vi "derive weighted array 2.vi"(10 "Full transition sequence from service to end":string[](array[string])=["0 1 0", "0 -1 0", "0 2 0", "0 4 0", "-4 1 0", "0 -4 0", "0 -2 0", "1 0 4", "1 -4 0", "0 -3 3", "0 -3 0", "1 -1 0", "-2 2 0", "0 1 -4", "2 0 -3", "0 -3 3 0", "-1 0 -1", "0 -1 1", "2 -1 0", "0 2 -1", "-3 0 1", "0 1 0 4", "1 0 4 0", "-3 3 0", "1 0 -3", "3 -2 0", "2 0 -3 0", "1 0 -1", "-4 0 -1", "0 -4 1", "2 0 -1", "0 -2 2", "-4 0 -3", "0 -1 1 0", "0 2 0 -3", "3 -3 0", "-4 0 1 0", "-4 1 -4 0", "-4 1 0 4", "0 1 -4 0", "-4 1 -4", "0 2 -1 0", "1 0 3", "0 -3 4 0", "-2 0 2", "1 0 1", "4 0 2 0", "0 2 0 3", "0 -1 2", "-1 0 -4", "1 0 -4", "0 -1 0 -1", "-1 0 2", "-1 0 -1 0", "1 0 -2", "0 -4 0 -1", "0 -2 2 0", "-1 0 1", "2 0 2", "0 1 -1 0", "0 3 -3 0", "-4 0 -2", "0 4 -4", "0 -4 0 -3", "0 4 0 1", "0 -2 0 2", "0 4 0 2 0", "-3 0 1 -4 0 -3", "2 0 1 0", "-2 0 2 0", "0 3 -2 0", "-3 3 0 -2 0", "3 -3 0 1", "-3 0 1 0", "4 -4 0", "0 4 -4 0", "0 -3 3 0 -2", "2 0 2 0", "-2 0 -1", "0 -4 0 1 0", "2 0 -4 0", "2 0 -1 0", "-1 3 -2", "2 0 1", "1 0 -3 3 0", "-4 1 -1", "-4 1 -1 0", "-1 0 -3", "3 -2 2", "-1 1 -1 0", "2 0 4", "1 0 -1 0", "0 -1 2 -1", "0 2 0 -2", "-3 0 -4 1", "0 1 0 -1", "-1 3 0", "0 -1 0 -4", "-2 0 -1 0", "4 0 4", "-4 1 0 4 0", "-4 0 -2 0", "-4 0 2", "0 -2 0 2 0", "0 2 0 -4 0", "2 0 4 0", "4 0 -2", "0 1 0 -4 0", "3 0 1", "2 -2 0", "4 0 -2 0", "0 2 0 4", "1 -4 0 1 0", "0 2 0 -2 0", "-2 2 0 -1 0", "-2 2 0 -1", "-1 0 4 0", "-2 0 4", "-4 1 0 3", "0 -3 0 1", "-2 2 0 -3 0", "0 1 0 3", "0 2 0 1", "0 1 0 1 -4", "0 1 -4 1", "-4 1 0 -3", "1 0 -3 0", "-3 0 -2", "2 -1 0 -1 0", "-3 3 0 -2", "1 0 4 -4 0", "0 -4 0 -3 0", "0 -4 0 1 0 -3 3 0", "0 -3 3 0 2 0 -3 0", "0 -3 3 -3 0", "3 -2 0 1", "-4 0 3", "-2 0 1", "0 3 0", "0 -3 4", "-3 4 0", "-3 0 4", "0 3 -3 0 1 -4 0 -3 3", "0 -2 0 -1", "-4 1 0 -2", "-4 0 -2 0 -1", "-2 0 -4", "0 1 0 -2", "0 -1 0 2 0", "0 -2 2 0 -1", "0 -3 -1 3", "-4 -1 0", "0 -1 2 0", "0 -3 0 -4", "2 0 -3 0 -4", "3 0 -1 1", "-4 1 0 -1", "-1 0 -1 2", "-1 0 -4 0", "0 -4 1 -1", "-3 3 -2", "2 -1 1", "4 -3 0", "1 -4 4", "0 2 0 -1", "1 0 1 0", "4 1 0", "0 2 0 2 0", "-4 0 -1 -3", "1 -4 0 -1", "0 -4 1 -4", "-1 3 0 -4 1 -4", "2 -1 3", "1 -3 0", "-2 0 1 -4", "1 0 -1 1", "0 -3 0 -4 1", "0 2 -1 0 1 -4", "0 -1 3", "0 -4 0 -1 0", "0 4 0 -2", "0 -2 0 -1 0", "0 -3 3 0 -2 0", "0 1 -1 0 -1", "0 -1 0 1 -1 0", "-1 3 -2 2", "-2 2 0 1 0 -1", "0 1 -1", "0 4 0 1 0 4", "-3 0 -4", "1 0 4 0 4 0", "4 -4 0 -2", "4 0 2", "-1 2 0", "1 -1 0 -1", "4 0 1", "2 0 3", "0 2 0", "0 -1 0", "0 1 0", "0 3 0", "0 -4 0", "-2 2 0", "1 -1 0", "0 -2 0", "0 -1 2", "0 1 -1", "0 3 -2", "3 -2 0", "0 2 -2", "-1 0 3", "2 -1 0", "-1 0 -1", "-1 0 -3", "-2 2 -2", "2 0 1", "2 0 2", "0 -3 0", "3 -2 2", "0 1 -1 0", "0 -2 2", "-1 2 0", "2 0 -1", "2 -2 0", "3 -3 0", "0 -1 2 0", "0 -1 0 3", "0 -1 1", "0 2 0 1", "2 -2 2", "0 -4 4", "0 4 0", "2 0 3", "-2 3 -2", "2 -2 3", "4 -4 0", "0 1 0 -3", "0 3 0 3", "-1 0 4", "-3 0 -2", "-4 0 -2", "2 0 2 -1", "-1 0 2", "-2 0 -1", "-4 4 0", "0 2 0 -2", "-1 1 -1", "-1 1 -1 0", "-2 0 -2", "3 0 -4 0", "3 0 3", "0 1 0 3", "0 3 -3 0", "2 0 -2", "3 0 -2", "0 -3 3", "3 -2 2 -2", "-3 0 -2 0", "1 0 -3 0", "-1 0 2 0", "3 0 -4", "-1 0 1", "-1 0 -1 0", "0 -1 2 3", "-1 3 -2 0", "3 -1 3", "-2 0 2 0", "0 1 0 -3 0", "0 -4 0 -2", "1 4 -4", "0 -2 2 0", "1 4 0", "0 3 -2 0", "-2 0 -4 4", "-1 0 3 0", "0 2 0 -1", "0 2 -2 3", "4 0 -1", "-1 2 0 2", "1 -1 0 -3", "-2 0 2", "2 0 -4", "0 3 -2 2 -2 2", "0 2 -2 0", "4 0 -4 0", "0 3 0 3 0", "4 -3 0", "-3 4 -3 0", "0 4 -4", "3 0 -1", "-2 2 -2 0", "0 -2 3", "-2 0 3", "1 0 -3", "2 -2 2 0", "0 -3 4", "0 -1 1 -1", "0 4 1 4", "1 -1 0 -1", "1 4 -4 0", "-4 0 2 0", "-4 0 2", "0 -2 2 3 0", "0 -1 1 -1 0", "0 2 0 1 4", "4 0 1 0", "2 3 -2", "0 -1 2 3 -2", "0 -1 0 4", "-4 0 1", "-1 0 -1 2", "-2 0 -1 0", "0 3 0 -1", "3 -2 0 -1", "0 -4 0 -2 0", "2 0 -4 0", "0 -2 0 2", "-1 0 -3 0", "0 -3 0 -2", "2 0 -1 0", "0 -1 2 0 1", "0 -2 0 -4 4 0", "0 -4 4 0", "-1 -3 0", "0 -2 0 3", "2 0 -2 2", "-4 1 0", "-1 1 4", "-1 0 3 -2", "0 2 0 4", "0 -4 4 0 -1", "3 0 -2 0", "0 3 0 -2", "2 0 1 -1 0", "0 1 -1 0 2 0", "0 2 0 1 -1", "2 0 -1 2", "-2 3 0", "0 -1 0 2", "0 1 -1 0 -3", "2 0 1 -1", "-2 0 -1 2", "-1 4 0", "0 -4 1", "2 0 2 0", "2 -1 1", "4 -4 0 -1", "-4 0 -1", "-1 0 4 0", "2 0 2 -1 0", "0 -3 3 0", "-1 0 -3 3", "-1 0 1 -1 0", "0 3 0 -4", "-2 2 -2 0 -2", "-2 0 4 0", "0 1 0 3 0", "4 -3 0 -2 0", "0 3 -2 3", "2 0 3 -2", "3 -2 3", "0 2 -2 3 -2 2", "-2 2 0 3", "3 -2 2 0", "3 -2 2 0 3", "3 -2 3 -2", "0 -3 4 -3 0", "0 -1 0 -3", "3 -3 0 1 0", "0 2 0 3", "0 3 -2 2 -2 2 0", "0 2 0 2", "-2 3 -2 0", "4 0 -2", "-4 0 -1 0 3", "-2 2 -2 3", "0 -1 0 -1 0", "-2 2 0 3 0", "0 2 -2 2", "2 3 -2 2 0", "-2 2 -1", "-4 0 -2 2", "0 -4 0 2", "-1 2 -1", "-1 0 3 -1 3 0 -4", "-1 3 -2", "4 0 -4", "3 0 3 0", "0 3 0", "0 1 0", "0 2 0", "0 4 0", "0 4 -4", "0 -3 4", "0 -3 0", "0 -4 0", "0 3 -2", "0 -1 0", "-4 1 0", "1 0 3", "0 2 0 -3", "2 0 3", "3 -3 0", "-3 0 3", "0 -3 3", "0 -3 4 -3 0", "0 -2 0", "3 -2 0", "0 3 0 1 0", "0 -3 4 0", "2 -2 0", "-2 0 -3", "4 0 2", "-3 0 2", "0 3 -3 0", "4 -4 0", "0 -1 2", "3 0 4", "0 3 -2 0", "0 -3 0 3", "1 0 -1", "0 4 -4 0", "-2 0 3", "0 2 -2 0", "0 2 0 -3 4", "3 -3 0 -3", "4 0 2 0", "3 0 -2", "0 -3 3 0", "-1 0 3", "0 -1 2 0", "-4 0 -1", "2 0 3 0", "0 3 0 3", "-4 0 3", "0 4 -4 1", "4 0 -3", "0 -1 0 4", "0 3 -3 0 2", "0 -2 0 3", "0 -3 4 0 3 0", "-3 0 4 0", "0 3 0 3 0", "0 4 0 -3 0", "-3 4 0", "2 0 -3 4", "0 2 0 -3 4 0", "0 1 0 2", "0 -2 3", "-2 0 -2", "0 -3 4 0 2", "0 -3 3 0 -2 2", "1 0 -3", "0 -1 1 0", "4 -4 0 -4", "-4 0 3 0", "2 0 -3", "-2 0 3 0", "0 4 -4 1 0", "-4 1 0 -1 2 0", "3 0 4 -4", "0 -3 4 -3 0 2", "3 0 3", "-1 0 -3", "-3 4 -3", "4 -3 0", "0 -3 4 -3", "-3 4 -3 0", "4 0 2 0 3", "0 2 0 3", "-4 1 0 -4 0 4 -4", "-4 1 -1", "-1 0 -4 0", "1 0 3 -2", "0 -1 0 3", "0 3 0 4 0", "0 2 0 3 0 1 0", "-4 1 -4 1", "1 -4 1 0", "0 -4 4", "0 1 0 4", "1 -4 1", "-3 0 1", "0 4 -4 0 -1 0", "-3 0 4", "2 0 -3 4 0", "1 0 2", "4 -3 0 2", "-3 4 -3 0 2", "3 0 1", "1 -1 0", "0 -1 0", "0 1 0", "0 1 -1 0", "0 4 0", "0 3 0", "-1 0 4", "-1 0 -3 3", "1 0 1", "-4 1 -1", "0 4 0 2", "0 -1 0 -3", "3 -2 2 -1 0", "2 -1 0", "0 1 -1", "-1 0 3", "-1 1 -1 0", "-3 0 1", "-1 0 3 0 -4", "-1 0 -3", "1 -1 0 -3 3", "1 -1 0 3", "2 -1 0 4 -4", "1 0 1 0", "0 -1 0 4", "2 0 3 0 -1", "-4 1 -1 0", "0 3 0", "0 -1 0", "0 4 0", "-1 0 3", "0 -3 4", "0 -3 3", "1 -1 0", "0 3 -2", "0 2 0", "0 1 -1", "4 -3 0", "-4 0 -3", "0 -4 0", "4 0 2", "0 1 -1 0", "0 1 0", "0 4 -4", "3 -2 2", "2 -1 0", "0 -2 0", "0 -3 4 0", "-1 0 -3", "0 3 -2 0", "0 -3 3 -3 0", "0 -3 4 -3 0", "4 0 4", "0 1 -1 0 3", "3 -2 2 0", "-2 2 0", "3 0 1", "0 4 0 2", "0 2 -1", "2 0 4", "-1 0 4", "0 -3 3 0", "-1 0 1", "-1 0 -1 0", "-1 0 -1", "4 -3 0 2", "0 -3 0", "-4 0 -3 0", "-3 0 3 -2", "0 3 -2 2 0", "-4 0 -3 3", "0 3 0 -4", "2 0 4 -4", "0 2 0 4", "0 4 0 -4", "2 -1 0 1 -1 0", "0 2 -1 0", "-1 0 -3 3", "0 -4 4 0", "0 4 -4 0", "-4 0 3 0", "0 -2 3", "-3 0 -3", "0 -2 0 -3", "-3 0 1", "-2 3 0", "0 3 0 -2", "0 4 -3 0", "4 -3 0 2 0", "0 -3 4 -3 0 3 -2 2 0", "3 0 -3 4 -3 0", "-1 0 3 -2 3", "-1 0 3 -2", "0 1 0 3", "1 0 3", "4 -3 0 -2", "-4 0 -3 4", "-2 0 3 0", "2 0 2", "0 2 0 2 0", "-4 4 -3 0", "0 -4 0 -3", "3 0 3 0", "-4 0 -3 3 0", "4 0 3", "0 4 0 4", "4 0 4 0", "0 4 0 -4 0", "0 -1 0 -2", "4 0 2 0", "1 0 -3", "0 -4 1 -4", "0 4 -4 0 -3", "-2 2 0 4 -4", "0 4 -4 4 -4", "4 0 2 -2", "0 4 0 -2", "0 3 0 1", "4 -4 1", "4 0 2 -1 0", "0 -4 4 0 2", "-1 0 3 0", "0 3 -2 0 -1 0", "1 -1 0 4", "0 4 0 1", "-1 0 4 0", "1 0 3 -2 0 -1 0", "0 -4 0 3 0 -4", "-1 0 -4", "1 -4 0", "1 0 4 0", "0 -1 0 -1 0", "-1 0 -3 3 0", "0 -1 0 -1 0 -3", "-2 2 -1 0", "0 -1 0 3 -2", "2 -1 0 1 -1 0 3", "-2 3 -2 2 -1", "-2 2 -1", "0 -1 0 4", "3 0 1 0", "0 3 -2 0 -1 0 -1 0", "-3 4 0", "3 0 -1", "0 4 -3", "3 0 3", "-4 0 3", "4 -4 0", "0 -1 0 -1", "0 3 0", "0 -3 4", "0 -3 3", "0 3 -3 0", "0 2 0", "4 -3 0", "0 3 -3", "0 3 -2", "0 -3 4 -3 0", "-4 0 -3", "3 0 -3", "0 -4 0", "-3 0 -3", "0 -3 3 0 3", "0 -3 3 0", "0 -2 0", "-3 0 3", "3 -3 0", "3 0 3", "-3 4 0", "-4 0 -3 4", "-3 0 4", "0 -1 0", "3 0 -3 3", "-3 3 0", "0 3 -2 0", "0 -3 4 0", "1 0 -3 4", "0 -3 0", "0 -1 0 -3", "-3 0 3 0", "-2 0 3 -2", "0 1 0", "0 -2 0 3", "-2 0 -3", "0 3 0 -3", "3 0 3 -3", "3 -3 0 3", "-3 0 -3 3 0", "0 -3 4 -4 0", "0 2 0 -2", "-2 0 3", "0 3 -2 3 0", "-2 3 0 -3 3", "3 0 -1", "-3 0 -4", "1 -1 0", "-4 0 -2", "0 3 -3 0 4", "-2 3 0", "-1 0 3 -2", "-3 4 -3", "0 -3 4 -3", "-3 4 -3 0", "-3 3 0 3", "-2 0 2", "0 -1 0", "0 -2 3", "3 -2 0", "-2 3 -2 0", "0 2 0", "0 1 0", "0 4 0", "2 0 -1 0", "0 3 -2", "2 -2 3", "-2 0 2", "0 2 -2 0", "4 -3 0", "-3 0 -2 0", "0 3 0", "0 -3 -2", "-2 3 -2 0 3", "0 3 0", "0 -2 0", "0 1 0", "0 3 -2", "2 -2 0", "0 2 0", "3 -2 0", "0 -3 4", "0 4 0", "-2 0 -2", "0 -3 0", "3 -2 2", "1 -1 0", "0 2 -2", "-2 3 -2", "0 -1 0", "0 -4 0", "0 2 -2 0", "-1 0 3", "0 -2 3", "2 0 -2", "0 3 -2 0", "0 -3 4 0", "-3 0 3", "0 3 -3", "4 -3 0", "-2 0 -3", "0 -2 3 -2", "-2 2 0", "0 3 -2 2", "3 -2 2 0", "2 0 2", "3 -3 0", "2 0 3", "0 -2 0 -2", "-3 4 0", "0 3 -3 0", "-1 0 3 0", "-2 0 1", "2 -1 0", "0 -3 4 -3", "0 3 -2 2 0", "-2 0 1 0", "-3 0 4", "0 -2 2", "-2 3 -2 0", "0 3 -2 3", "0 1 -1 0", "1 0 1", "0 -3 0 3", "0 -3 3", "3 0 -3", "0 -1 0 3", "4 0 1 0", "0 -2 3 -2 0", "2 0 3 -2 0", "0 2 -1", "3 -3 0 4 0", "-2 0 -4", "-3 0 -2", "3 0 3", "0 3 0 3 0", "0 3 -2 3 -2", "-2 3 -2 2", "-3 0 1", "-2 0 3", "-2 0 -3 0", "0 3 -2 2 0 2", "2 0 2 0", "1 -1 0 3", "0 3 -2 0 -2 2", "-2 0 -2 2", "2 0 -2 3 -2", "1 0 -2", "1 0 3", "2 0 -4 0", "-1 0 1", "0 2 0 4", "4 0 -2", "0 -2 0 1", "0 -1 0 3 0", "0 2 0 3 -2 0", "0 3 -2 0 1 0", "-1 0 -1 0", "-2 2 0 -2", "2 0 -2 0 -2", "0 4 0 1 0", "0 1 0 4 0", "0 1 0 -3", "0 -3 0 3 -2", "1 0 -3 0", "4 0 -4 0 1", "-1 0 -4", "0 -3 3 -3 0 4 0", "0 -4 0 3", "0 3 0 2", "1 0 1 0", "0 4 0 3", "1 -1 0 -3 4 0", "3 -2 0 -4", "2 -1 2 0", "-4 1 0", "3 -2 0 -4 0", "-2 0 -3 4", "0 -3 4 -3 0", "0 -2 0 -3", "-2 0 -3 4 -3 0", "2 -2 3", "0 2 -1 0", "2 0 2 -2 0", "0 -3 4 0 2", "1 0 2", "-3 4 0 2 0", "-2 0 -4 1", "0 3 -2 0 -4", "0 2 0 2", "-2 3 0", "1 0 -3", "0 3 0 -3 4", "-3 4 0 2", "-2 0 -2 2 -2 0", "2 -2 0 -3 4", "0 -3 4 -3 0 3", "4 -3 0 3 0", "3 0 -2", "0 -2 0 -2 0", "4 -3 0 3", "0 4 -3 0", "-3 0 -2 0", "-1 0 -1", "1 0 4", "2 0 2 -2", "-2 0 -2 0", "1 -1 0", "-1 0 1", "0 1 0", "0 -1 0", "0 1 -1", "-1 0 -1", "0 4 0", "2 -1 0", "-1 0 1 -1", "-1 0 4", "0 -3 0", "0 1 -1 0", "-1 1 -1", "-1 0 -3", "-1 0 -1 0", "0 -1 0 1", "1 -1 0 -1", "-1 1 -1 0", "1 -1 1", "4 0 2", "0 1 -1 0 1", "1 -1 0 4", "0 1 0 -4", "0 4 -4", "-1 0 -1 0 1", "-1 0 4 0", "0 1 -1 1 -1 0", "1 0 -4 0", "1 0 -4", "0 4 0 -1 0", "-1 0 1 0", "0 4 -4 0", "-1 0 -3 4 0", "0 1 0 -1 0 -3", "0 1 0 -4 0", "-4 0 4", "0 -1 1 -1", "-2 2 -1 0", "0 -3 0 -1 0", "2 -1 0 -3", "-1 0 3 0", "-1 0 -3 0", "-1 0 -2", "0 2 0", "1 -1 0 4 0", "-1 0 4 0 -1 0", "0 1 -1 1 -1 0 4", "0 -2 2 -2", "-1 0 -1 0 1 0", "3 0 1 0", "0 4 0 1 -1", "1 -1 0 1", "0 1 -1 1", "1 -1 1 -1", "0 1 -1 1 -1", "1 -1 1 -1 0", "0 -1 1", "0 -4 0", "-3 0 -1", "4 0 -1", "-1 1 -1 0 4", "1 -1 1 -1 0 4", "-2 2 0", "1 -1 0", "0 1 0", "0 -1 0", "3 -3 0", "0 3 0", "0 1 -1", "0 4 0", "0 2 0", "2 -1 0", "-1 0 1", "0 -2 0", "-4 1 0", "1 0 1", "0 1 -1 0", "-1 0 -3", "-1 0 4", "0 4 0 -2", "0 4 -4", "-1 0 1 0", "0 3 -3 0", "0 -4 1", "0 4 -4 1", "-4 4 0", "-1 0 3", "0 -2 3", "0 -3 4", "1 0 1 -1", "-2 0 -3", "0 -3 0", "0 -3 3", "-2 3 -3 0", "1 0 -2", "-2 3 -2", "4 -4 1", "1 -1 0 4 -4 1", "-1 0 4 -4 1 -1", "-4 1 0 1 -1 0", "0 1 0 -4", "0 1 0 -2", "-1 0 -1 0", "2 -1 0 1", "1 -1 0 1 0", "3 -2 0", "0 -2 2", "2 0 2", "3 -3 0 1", "-3 0 3", "-2 2 0 -3", "0 3 -3", "-3 0 -4 4", "0 4 0 -2 3", "0 -4 4", "-1 0 3 0", "4 -4 1 0 4", "4 0 1 0", "1 -1 0 -3", "-2 0 1 -1", "0 4 -4 1 0", "0 -4 4 0 1", "1 0 -2 3 -2", "1 0 4", "0 -4 1 0", "0 1 0 -4 1 0", "-2 0 1", "4 -3 0", "-3 0 4", "0 4 -3 0", "1 -1 0 4 -4 1 -1 0", "4 -4 1 0", "1 0 4 0", "1 -1 0 -1 0", "0 -4 0", "4 0 1", "0 1 0 1 0", "2 0 4 0", "0 -2 0 2 0", "2 0 1", "-1 0 -3 4", "4 0 2 0", "0 -2 0 1", "-1 0 4 -4 1", "3 -2 3", "3 -2 2 0", "1 -1 0 3", "-1 0 -1", "0 -1 1", "-1 0 1 0 3", "0 -4 1 0 1 -1 0", "0 3 -2", "0 1 0 3", "1 -4 0", "0 -2 2 0", "1 -1 1 -1 0", "0 1 0 3 -3 0", "-3 0 -3 3", "0 -3 3 0", "0 3 0 -2 0", "0 2 0 2", "-4 0 -2", "3 0 3", "3 0 3 0", "0 -3 3 -2", "0 2 -2 3 -3 0", "-2 2 0 -3 3", "-3 0 1", "3 -3 0 3", "0 3 -3 0 1", "0 3 0 2", "2 0 -3", "-2 3 -3", "3 -2 2", "-4 1 -1", "2 0 -3 3", "0 4 0", "0 -2 0", "1 -1 0", "-1 2 -1", "0 2 0", "2 -1 0", "0 3 0", "0 -1 0", "-2 0 3", "0 -4 0", "3 -2 0", "0 3 -2", "0 -3 0", "-1 0 3", "0 -2 0 3", "0 1 -1 0", "0 3 -2 0", "1 -4 0", "-1 0 2", "0 -1 2", "2 0 3", "0 -3 3", "3 -3 0", "3 0 -1 0", "-2 0 -2", "2 -2 0", "-3 3 0", "0 2 0 3", "0 1 0", "0 -2 2", "-4 0 -1", "0 -1 2 -1", "-1 0 -1", "2 -1 2", "-1 3 -2", "3 0 -4", "3 -2 2", "-1 1 -1 0", "-1 2 -1 0", "0 1 -4", "4 -4 0", "2 -3 0", "0 3 0 -2", "2 0 3 0", "0 1 0 -3", "1 0 -3", "-1 0 -4 0", "-4 0 1", "2 0 -2 0", "-1 0 -3", "0 -3 4", "4 0 1", "0 1 -4 0", "0 -1 0 3", "0 -3 3 0", "0 3 -3 0", "0 4 0 2", "0 2 -2 0", "-2 0 -3", "3 0 3", "-1 0 -2", "-2 0 3 0", "2 0 4 0", "0 4 0 -2 3", "0 -3 0 -2", "-3 0 -2 2", "1 0 4 0", "-3 0 2", "0 -2 0 3 -2 0", "1 0 -3 0", "-3 0 -2", "-2 0 -2 0", "0 4 -4", "-1 -3 0", "-2 2 -1", "2 0 -3", "-1 1 0", "2 -1 1", "-2 2 0", "0 -4 0 -1", "0 -1 3 -2 2", "-1 2 -1 2", "-1 2 0", "-1 3 0 -1 0", "2 0 2", "-1 0 2 -3 0", "-1 0 2 0", "-1 4 -4 1", "-1 0 4", "2 -1 0 -1", "2 -1 0 2", "-4 1 -1", "3 0 -4 1", "1 -1 -3 3", "0 1 0", "0 -2 0", "1 -1 0", "0 3 0", "0 2 0", "0 3 -2", "3 -2 0", "0 -4 0", "-1 0 -2", "-2 2 0", "0 -1 0", "1 -1 0 -2", "0 -2 2", "-2 0 -2", "0 1 0 1", "4 -4 0", "0 3 -3", "0 1 -1", "1 0 1", "0 3 -2 0", "-2 2 -2", "0 -2 3", "0 3 -3 0", "0 4 0", "2 0 3", "0 -2 3 -2", "0 4 -4 0", "-2 0 -2 0", "1 -1 0 -2 0", "-2 0 2", "-4 0 -4", "0 -4 0 1", "0 2 0 -4", "3 0 -2", "-1 0 3", "0 1 -1 0", "-3 0 -1", "-1 0 2 0", "4 -3 0", "1 0 -2", "0 1 0 1 0", "0 -2 3 -2 0", "3 -2 0 -2 0", "0 -2 2 -2 0", "0 -2 0 -2", "-1 4 0", "4 0 2", "1 -1 0 -2 0 2 0", "2 0 -2", "-2 0 4", "0 -1 0 3", "0 -2 2 0", "1 0 3", "0 1 0 3", "4 0 -2", "0 -4 0 -4", "0 2 0 -4 0", "-4 0 -4 0 1 0", "-1 2 3 0", "3 0 3", "0 -4 0 3 0", "2 0 1", "2 -1 0", "-1 0 -1", "-2 3 0 -2", "3 0 -2 0", "0 1 -1 0 -2", "0 3 0 -2", "3 -2 2 -2", "1 0 1 -1", "0 4 -3 0", "2 0 -1 0", "0 2 0 3", "2 0 3 0", "2 0 -3 4 -3", "-2 2 0 -3 4", "2 0 -3 4", "0 3 -3 0 -1 0", "1 0 4", "0 3 0 1", "1 0 3 -2 0", "-2 3 0", "1 0 1 0", "0 4 0", "0 2 0", "0 3 0", "0 -3 0", "0 1 0", "-4 0 -3", "0 -4 0", "0 3 -3 0", "0 -3 0 3", "-4 0 3", "0 4 0 2", "0 -3 3", "-4 0 -3 0 3", "0 2 0 3", "-3 0 2", "0 4 0 1", "0 -4 0 3", "0 4 0 2 0", "0 -2 0", "0 1 0 4", "4 0 2", "0 4 0", "0 3 0", "0 2 0", "4 -4 0", "0 4 -4 0", "0 -2 0", "3 -3 0", "0 4 -4", "0 3 -3", "0 3 -2", "0 4 0 2", "4 0 2", "0 1 0", "0 3 -3 0", "0 -3 0", "2 -1 0", "0 -1 0", "1 0 3", "4 0 3", "3 -2 0", "0 1 -4", "-1 0 4", "0 -4 0", "0 -3 3", "2 0 4", "-4 1 0", "0 -2 2", "0 4 0 3", "-1 0 1", "0 3 -2 0", "-3 0 4", "-1 0 3", "0 -3 4", "0 4 0 -2", "1 -1 0", "2 0 4 0", "0 -4 4", "0 -1 0 4", "-1 0 4 0", "4 -3 0", "0 2 -1 0", "1 -4 0", "2 0 -4", "-2 0 4", "0 4 0 2 0", "3 0 3", "0 -3 3 0", "2 -2 0", "1 0 -3", "-4 0 2", "1 0 3 0", "0 1 0 3", "-1 0 3 0", "3 -2 2", "-4 1 -1", "2 0 -3", "0 -4 1", "0 2 0 -4", "-3 0 4 0", "3 0 -2", "0 -2 2 0", "0 -2 3", "-4 0 2 0", "0 3 0 -4", "0 2 0 4 0", "-2 0 2", "-2 2 0", "0 3 0 4", "-3 4 0", "-1 0 1 0", "4 0 4", "0 1 0 3 0", "0 -1 0 4 0", "0 3 0 3", "1 0 -3 0", "0 3 0 1", "-2 2 -1 0", "0 3 -2 2", "-3 0 2", "1 -1 0 3 0", "0 3 0 -2", "-4 0 -4", "0 1 0 -3 0", "0 4 0 -3", "2 -1 0 4", "1 -4 1", "-4 0 3", "-2 0 -4 0", "0 3 -3 0 4", "-4 0 -2", "0 4 -4 0 3", "0 -2 3 -2 0", "0 4 0 4", "-1 2 -1", "-3 0 -2", "-3 0 -3", "-4 0 4", "4 0 -3", "3 0 -4", "2 0 -2", "-2 0 2 0", "0 -4 4 0", "0 2 0 3", "-2 0 1", "4 0 3 -3 0", "0 -2 0 3", "0 4 0 3 0", "0 2 -2 0", "2 -2 0 4", "4 0 -2", "2 0 -1", "0 1 -4 0", "0 -1 2", "4 0 -1", "0 1 -4 1", "4 -4 1", "0 3 -2 0 1", "4 0 4 0", "0 -1 0 4 0 4", "1 0 4", "0 1 -4 1 0", "0 4 0 2 0 -3", "-2 0 4 0", "0 2 -2 0 4 0", "0 -3 0 2", "-4 0 -2 0", "0 -2 0 2 0", "0 2 0 -1", "0 -1 3", "0 -4 4 -4", "3 -2 0 -4 0", "-4 0 -1", "-3 0 3 0 3", "-1 0 3 -3 0", "-3 0 3 0", "0 3 0 3 -2", "-2 2 -2", "-1 0 1 0 3", "-2 2 -1 0 1 0", "0 2 -1 0 -3", "0 4 0 2 -1 0", "-1 0 4 -4 0", "0 2 -1 0 4 -4", "0 4 -4 0 3 -2 0", "-1 0 -3", "-2 0 1 -4", "0 3 0 4 0", "0 1 -4 4", "-1 0 -3 0", "-1 0 4 -4", "0 4 0 -2 0", "0 4 -3 0", "4 0 -3 3", "-1 0 -2", "0 -2 0 3 -3", "1 -4 1 -1 0", "-4 1 -1 0", "-2 0 -2 2", "0 -1 2 -1", "-4 0 -4 1", "0 2 0 4 0 2 0", "0 3 0 -1", "3 0 3 0", "0 -3 0 3 0", "0 3 0 4 -4 1", "-1 0 -4", "0 -4 1 0 3 0", "0 2 -1", "-4 0 4 0", "0 -2 0 4", "0 4 0 -1", "-4 0 3 0", "0 3 0 -2 0", "0 -3 4 -3 0", "-4 0 2 0 -4", "2 0 -2 0", "-2 2 0 -3", "3 0 2 0 4 0", "3 0 2 0", "1 -4 0 2 0", "3 0 -4 4 0", "3 0 -4 4", "3 -3 0 4", "-2 3 -3", "0 -4 0 2 0", "0 3 0 -4 0", "3 -3 0 4 0", "0 3 -3 0 4 0", "4 0 3 -2", "-4 0 -3", "-3 0 -3 4", "3 -3 4 0", "1 -4 -1", "-3 3 -3 0", "0 -1 1", "-3 0 4 0 3", "0 3 -3 0 -2", "0 4 0 3 -3 0", "4 -3 0 4", "0 3 0 2 0", "0 4 0 -2 2", "-4 -1 0 1", "-1 0 1 0 -3 0", "-3 0 1 -4 0", "-3 3 0", "0 -1 0 1", "-1 0 1 -4", "0 3 0 -4 4", "-4 1 -1 0 3 0", "0 1 0 3 0 1", "-3 0 3", "4 0 -2 0", "4 0 2 0", "3 0 -1", "4 0 3 -3", "3 -3 0 -2", "3 0 4", "3 0 2", "2 0 3", "4 0 -2 2", "-2 2 -1", "0 2 -1", "0 4 0", "2 -1 0", "0 -4 0", "0 2 -1 0", "3 -2 0", "4 -3 0", "0 -1 2 0", "0 -1 0", "0 2 -2", "-4 0 1", "-4 0 -4", "0 -4 0 -4 0", "-1 0 4 0 2", "-2 2 0", "1 0 -4 0", "3 -2 2", "0 2 3 -2", "2 -1 0 2 -1", "2 -1 -3", "3 -2 0 -4", "0 -3 4 -3 0", "-1 1 -1 0 -1", "0 -4 1 0", "-1 0 2", "4 0 2", "0 2 0", "0 1 0", "0 -4 0", "0 -2 0", "0 2 -2", "2 -2 0", "0 4 0", "0 3 0", "0 2 -2 0", "0 -1 0", "0 -3 0", "-4 0 -2", "-2 0 2", "1 0 4", "-2 0 -4", "0 3 -2", "3 -2 0", "1 -1 0", "-2 3 0", "0 -1 2", "0 -3 4", "4 -3 0", "-2 0 4", "0 4 -3", "-2 0 -4 0", "-2 2 -2", "3 0 1", "4 0 2", "-1 0 -1", "0 -2 3", "1 0 -4", "-1 0 -1 0", "-2 0 -3", "1 0 -3", "-2 0 3", "2 0 -2", "-2 2 -2 0", "-4 0 -2 0", "0 1 0 4", "0 3 -3", "2 0 1", "1 -4 0", "0 -4 1", "0 3 -2 0", "-3 4 0", "0 -4 0 -2", "2 -1 0", "0 3 0 1", "0 1 -4 0", "3 0 2", "-3 0 -4", "-4 0 2 -2 0", "0 -4 0 2 -2", "2 0 -2 0", "0 4 -3 0", "-4 0 2", "-4 0 2 -2", "-2 2 0", "-4 1 0", "0 4 -4", "-2 0 2 0", "0 -2 0 2", "1 0 3", "-2 0 4 0", "2 0 -4", "-2 3 -2", "0 2 0 1", "0 4 0 2", "0 2 -2 2", "0 1 -1", "0 -4 0 -3", "-1 0 -4", "-1 0 -2", "2 -2 0 -4 0", "2 0 3", "0 -4 0 2", "0 -3 4 0", "0 3 -3 0", "0 -4 0 -2 0", "-2 0 -2", "0 -3 3", "0 -2 0 -4", "0 -4 1 0", "4 0 2 -2", "-3 0 -4 0", "0 -3 4 -3 0", "2 -2 0 2", "0 1 0 -1", "2 -2 0 4 0", "2 -2 0 4", "1 0 -4 0", "-3 0 3 0", "0 3 0 -2", "2 -2 3", "0 2 0 -2 0", "0 1 0 3", "1 0 4 0", "-4 4 -4 0", "-2 0 1", "0 -4 0 3 0", "1 0 1 0", "-1 0 3", "0 -1 2 -1", "0 -1 0 -1", "0 4 0 3", "0 -2 0 4", "0 -4 4", "0 3 0 1 0", "1 0 -3 3", "0 2 -1", "-1 0 1", "-2 0 -3 0", "1 -1 0 -2", "-1 0 -2 0", "3 0 3", "-1 1 0", "3 0 -2", "3 0 4 0", "0 2 -2 2 -2 0", "0 1 0 -4", "0 2 0 4 -3", "-2 0 -2 0", "0 3 0 -2 0", "-2 0 -2 3", "0 2 0 3", "0 -2 0 2 0", "0 -3 3 0", "4 0 -3", "0 1 0 -3", "1 0 4 -3 0", "2 -2 0 -2", "0 -1 1", "-1 1 -1 0", "0 1 0 -1 1", "0 -3 0 -3", "-1 0 -3", "4 -3 0 1", "-3 4 0 2", "0 2 -2 0 -3 4", "3 -2 0 -3 0", "0 -2 0 3", "-2 0 -4 0 2", "0 2 -2 0 -4 0", "0 -2 0 4 0 3", "4 0 -2 0", "0 -4 0 -3 4", "0 1 0 -4 0", "0 -2 2", "0 4 0 4", "2 0 -4 0", "-4 0 -1 2", "3 0 3 0", "0 3 0 2", "0 2 -1 0", "2 -2 3 0", "0 1 -1 0", "0 1 0 4 0", "0 1 -4 0 -2", "0 -2 0 2 -2 0", "0 -2 0 -3", "-4 0 1", "-2 0 2 -2 0 3 0", "-2 0 3 0 1 -4 0", "4 -1 0", "0 2 -2 0 2", "2 0 2 -2", "1 0 -4 4", "-1 0 4", "2 -1 0 -4 0 -3", "0 -1 2 -1 0", "-1 0 3 0", "-3 0 3 0 1 0", "1 -4 0 -4", "0 1 0 -2", "-2 0 -4 0 3 0", "0 4 0 2 -2 2 -2 0 -4 0 3", "0 2 -2 0 4", "-2 0 2 -2 0", "0 -1 1 0", "1 -1 0 -2 0", "0 -4 0 3", "4 0 1", "-2 0 -1", "-1 0 -1 0 -1", "0 1 0 3 0", "-1 2 0", "-1 0 1 0", "3 -2 3", "0 -2 3 0", "3 0 2 0", "0 3 0 4 0", "-1 0 2", "0 -3 0 -1 0", "-4 0 -3", "-1 0 -2 3", "0 -2 3 -2", "0 -2 3 -2 0", "-2 0 -4 0 3", "0 3 0 3", "0 -2 0 -4 0", "0 4 0 -4 0", "1 0 2", "3 0 -2 3 -2", "-3 0 2 -2 0", "4 -3 0 2", "-3 0 -2 0", "2 0 4", "0 2 0 4", "2 0 4 -3", "0 2 0 4 -3 0", "-3 0 2", "-3 0 -3", "4 0 4", "1 0 -2", "-2 0 2 -2", "1 0 1", "2 0 4 -3 0", "-3 0 3", "3 -3 0", "0 3 0", "-3 3 -3 0", "-3 3 -3", "0 -3 3 -3", "0 -3 3 -3 0", "2 -1 0", "0 -3 3", "-3 0 -3", "3 -3 0 -3", "-3 0 -3 3", "0 2 -1", "0 1 0", "0 3 0 3", "0 -1 0", "3 -3 0 -3 3", "0 2 -1 0", "0 4 0", "0 3 -2", "-1 0 2", "3 -2 0", "0 -4 0", "0 -3 0", "3 0 2", "0 3 -3", "0 -3 4", "-3 0 -3 3 -3", "0 3 -2 0", "-1 0 4", "-1 0 3", "-1 0 3 0", "0 1 0 3 0", "1 0 -1", "0 1 0 -1 0", "3 0 1", "0 2 0", "0 -1 2 0", "-3 0 -2", "3 0 -3", "0 -2 3", "0 -3 3 -3 0 -3 3", "3 0 3", "0 2 -1 0 2", "0 2 -2", "2 -2 3", "1 -1 0 3", "0 3 -2 0 1 0", "0 4 0 -1", "0 1 -4", "2 -1 0 4", "0 4 -4", "0 1 0 3 0 1 0", "1 0 3", "0 1 0 3", "1 0 3 0", "2 0 -1", "0 -1 0 3 0 3 0", "0 2 0 3 0", "2 0 4 0 2", "-4 0 -3", "4 -4 0", "0 3 0 3 -3", "-4 0 3 0", "0 -3 4 -3", "-3 3 0", "-2 0 3", "0 -2 0", "1 0 -3", "2 -2 0", "3 0 -3 4", "-3 0 -3 3 -3 0", "3 -3 0 -3 3 -3 0", "0 -3 3 -3 0 -3 3 -3 0", "0 3 0 -3", "-3 3 -3 0 -3", "0 -3 3 -3 0 -3", "-3 3 -3 0 -3 3", "2 -1 0 2", "3 0 3 0", "2 0 3", "3 -3 0 -3 3 -3", "0 3 0", "0 2 0", "0 4 0", "0 -3 4", "0 1 0", "2 -1 0", "0 -1 0", "0 -3 3", "2 0 3", "0 4 -4", "1 -1 0", "0 3 -2", "3 0 3", "0 2 -1", "-4 0 -3", "0 -3 0", "-1 0 4", "-1 0 2", "4 -4 1", "4 -4 0", "0 -2 3", "3 -3 0", "0 1 -1", "0 1 -4 0", "3 0 3 0", "1 -4 0", "0 2 0 3", "3 -2 0", "0 3 0 3", "-1 0 3", "1 -1 0 4", "0 2 -1 0", "0 -3 4 -4", "3 0 1", "0 -2 0", "0 4 -4 0", "0 3 0 3 0", "1 0 3 0", "3 -2 2", "-4 0 -3 3", "3 0 -3", "0 -3 3 -3 0", "3 0 -2", "-4 1 0", "0 -4 4", "2 -1 0 -3", "0 3 0 1", "2 0 -3", "-3 0 1", "-4 1 -1", "0 2 -2", "-2 3 0", "1 0 1", "0 -1 0 2", "0 3 -2 2", "0 1 0 3", "0 -4 1", "0 -3 3 0", "-2 2 0", "-2 0 3", "1 0 4 0", "4 -4 1 0", "0 1 -1 2", "1 0 1 0", "0 1 0 1", "-1 0 4 -4", "2 -1 0 3", "1 -1 2", "-1 2 -1 0", "0 4 -4 1 -1", "0 -3 4 -4 1", "4 -4 0 -3 3", "0 -4 4 -4", "-1 0 2 -1", "-2 0 -1", "1 -1 0 4 -4", "0 4 0 3", "2 0 4", "4 -4 0 -3", "0 3 0 -2", "0 -3 4 0", "1 0 3", "-4 0 3", "-3 0 2", "0 3 -2 3", "0 2 0 3 0", "0 4 0 2", "4 -3 0", "-3 0 1 0", "0 2 0 -3", "0 1 0 3 0", "0 -4 0", "0 -4 0 -3", "2 -2 0", "2 0 -2", "0 3 -3", "2 -1 0 -3 4", "-1 0 -2", "1 -1 0 3", "-1 0 3 0", "0 -1 2", "0 -3 4 -4 1 0", "0 4 0 -1", "1 0 -3", "0 3 -2 0", "0 1 0 4 0", "0 4 0 -4", "0 4 0 3 -2", "3 -2 0 1 0", "2 -1 0 -3 0", "-3 0 -4", "0 4 -4 1 -1 0", "-1 0 4 -4 0", "0 4 -4 0 2", "-3 0 -1", "0 3 0 1 -1", "-1 0 4 0", "0 1 -1 2 -1 0", "2 -1 0 2", "0 2 0 -1", "-1 0 -1 0", "-1 0 2 -1 0", "0 1 0 2", "0 2 0 -3 4 -4", "1 0 3 0 2", "0 -2 3 -2", "3 -2 0 -1", "0 4 -4 0 -3", "1 0 -4", "-4 0 -3 3 -3 0", "-2 3 -2 0", "-2 3 -2", "0 4 0 2 0", "-4 0 3 0", "0 1 -4", "0 -3 3 0 -2", "0 -2 0 2", "-2 0 2 0", "3 0 -2 0", "-4 0 -3 0", "0 -3 0 3", "0 3 -3 0", "0 -3 4 -3 0 1 0", "0 3 -2 2 0", "2 0 2", "0 2 0 2 0", "0 3 0 -3", "3 0 -3 4", "0 1 0 1 0", "0 -3 3 -2 0 3", "0 -3 4 -4 0 -3 3 -2", "0 -3 0 2 0", "0 2 -2 0", "0 -3 3 -2", "2 0 -4 0 -3 3", "3 0 -2 3", "0 2 0 -2", "0 2 0 4 0", "-2 0 -2 3 0", "0 1 0 3 0 -2", "-3 3 -3", "0 -3 3 -3", "-3 3 -3 0", "1 0 4", "-4 0 2", "-1 0 -1", "3 0 2", "-3 4 -4", "4 0 3", "-2 0 2", "2 0 3 0", "0 2 -1 0 3", "-3 3 -2", "0 -1 0", "0 3 0", "-1 0 3", "0 3 -2", "-1 0 3 0", "0 1 0", "0 3 0 -1", "-1 0 -1", "3 0 -1", "0 -1 0 3", "-1 1 0", "-1 0 3 -2", "-1 0 -1 0", "0 -1 1 0", "0 -1 0 -1", "0 -1 1", "3 -3 0", "0 1 -1", "0 3 -3", "0 -1 0 -1 0", "0 -3 3", "0 -3 3 0", "0 3 0 3", "1 0 -1", "0 1 -1 0 3", "0 3 0 -1 1 0", "2 -1 0", "1 0 3", "0 3 -2 0", "0 3 -3 0", "0 -1 0 1", "0 2 -1 0", "-1 2 0", "0 1 0 -1", "1 0 -1 0", "0 -1 0 3 0", "0 -1 0 3 -2", "-2 2 0", "2 0 -2", "-1 0 3 -2 3 0", "0 -1 0 -1 0 3", "-1 0 3 -2 3", "-1 0 -1 0 3 -2", "0 2 0", "0 -3 0", "0 -1 2 0", "0 -1 0 -1 1 0 3", "0 -1 0 1 -1 0 3 -2", "1 -1 0 3 -2 3", "2 0 3", "0 3 -3 0 3", "0 -3 3 0 1 0", "1 -1 1 0", "0 3 -2 2 0", "3 0 3", "1 0 -3", "-1 1 0 1", "3 0 1 0 3", "0 -1 0 2 -1 0", "-1 0 -3 3 0", "3 0 1", "3 0 1 0", "0 -2 2", "-1 0 3 0 -1", "0 3 -2 0 -1 0", "3 0 -1 1", "1 -1 0 3 -2", "-1 0 3 -2 0", "0 3 0 -1 1", "3 0 -1 1 0", "-2 -1 0", "-1 0 -1 0 3", "0 -4 0 1 0", "3 0 -1 0", "3 0 -1 0 3", "1 -1 0 3", "1 0 3 0", "0 3 -2 0 1", "0 1 0 -1 0", "0 1 -1 0 3 0", "3 -2 0", "-1 0 1", "1 0 1", "1 -1 0", "0 -1 0", "-1 0 -1", "0 -1 0 -1", "1 -1 0", "0 1 0", "-1 0 3", "2 -1 0", "0 3 0", "0 -1 1", "-1 0 -2", "-2 2 -2", "-1 0 -1 0", "3 -3 0", "0 -2 0", "0 1 -1 0", "-2 0 -1", "0 3 -2", "-2 0 -1 0", "4 -3 0", "0 -1 1 -1 0", "0 -1 0 -1 0", "0 -1 0 3", "-3 0 1", "-1 0 3 0", "3 0 -1", "2 0 3", "0 2 0", "-1 0 -3", "0 -2 3", "0 -1 0 -2", "0 -1 0 -1 1", "0 2 -1", "-1 0 3 -2", "0 1 0 3", "-2 2 -1 0", "2 0 -1", "3 -3 0 1", "-1 0 1 0", "-2 2 0", "3 -2 0 -1 0", "-1 0 2", "0 2 -1 0", "1 0 1", "0 -4 0", "0 4 -3", "0 4 -3 0", "0 -1 0 -3", "0 -3 3 -3 0", "-2 2 -2 0", "-3 0 4", "0 3 -2 0 -1 0", "0 1 0 3 0", "0 3 -3 0", "2 -1 0 2", "-1 0 2 -1", "1 -1 0 -2", "-1 0 1", "3 -2 2", "0 -1 1 0", "-1 0 -2 2", "0 3 0 -1", "-3 0 1 0", "0 -1 0 3 0", "2 -2 0", "0 -3 0", "0 2 0 3", "3 -3 0 1 0", "1 0 -2", "-2 3 0", "-2 0 -2", "2 0 -1 0", "0 -1 0 1", "0 -1 2", "2 0 3 0", "3 0 -2", "0 2 0 -1", "-3 0 2", "-1 0 -2 3", "3 0 -1 1", "3 0 -1 1 -1 0", "0 2 3", "1 -1 0 3", "3 -2 2 -1 0", "-2 2 -2 2", "0 -1 0 -2 2", "-1 0 -1 0 -1", "0 -1 0 -1 1 -1 0", "2 -2 3", "-1 0 -1 0 -2", "-1 0 -2 0", "3 0 1", "0 3 0 1", "-1 0 3 -2 0 -1 0", "0 3 -2 2 -1 0", "0 1 0 -1 0", "3 0 1 0", "2 -1 0 -1", "0 -2 0 -1", "0 1 -1 0 -2 3", "-4 0 1", "0 2 0 -1 0", "-1 0 3 0 -1", "3 0 -1 0", "0 3 0 3", "3 -3 0 2", "-3 0 1 0 1", "0 3 0 -3", "-3 0 3", "4 -3 0 3", "-2 2 -2 0 -2", "2 -2 0 -2 0", "-1 0 -3 3 -3 0", "1 -1 0 -3", "0 -1 0 1 0", "0 -3 -2 3 -3 0", "-2 0 2 0 3 0", "3 0 -2 0", "0 -2 0 1", "0 -1 0 -3 0", "0 3 0 -1 1 -1 0", "-2 2 0 -1", "2 0 -1 1", "3 -2 0 -1 0 -3", "0 3 -3 0 1 0", "0 -3 3 -3 0 1", "0 -2 3 0", "2 -2 0 -2", "-3 0 1 -1 0", "-1 2 0 3", "0 -1 0 -1 1 -1 0 -2 0", "-2 2 -1 0 3", "-2 2 -1 0 3 -2", "2 3 0", "0 -1 0 2", "-1 3 0", "3 0 2", "3 -1 3", "-2 3 0 -1 1", "-2 3 0 -1", "0 -1 0 -1 0 -2", "0 -4 1", "-4 1 0", "0 -1 1 0 -2 0", "0 -2 3 -2 2", "3 -2 2 -1 0 3", "2 -2 3 0 -1", "1 -1 0 -1 0", "1 0 2", "-1 0 -4", "2 -1 0 -1 0", "-1 0 -1 1", "0 3 -2 0 -1 0 -1 0", "1 -1 0 3 -2 0 -1 0 -1", "0 -1 0 -1 0 -1 1", "0 1 0 3 -2", "0 -1 0 -1 1 0", "0 -1 0 3 -2 2 -1 0", "1 0 1 -1 0", "3 -2 0", "3 -2 0 -1", "-2 0 -1 0 3", "0 1 -1", "0 3 0 1 0", "3 0 -3", "2 -2 2", "-2 0 -1 0 -1", "3 -2 0 -1 0 -1", "0 -2 2", "0 3 -2 0", "0 3 -2 0 -1", "1 0 3", "-1 1 0"]) -> (1 "weighted array (NON directional transitions)":dbl[][](array[numeric]), 2 "weighted array (directional transitions)":dbl[][](array[numeric]), 3 "weighted array positions only":dbl[][](array[numeric]))   [LabVIEW 2014]
panel:
  out "Position weights 3":i32[](array[numeric])
  out "averaged position weights 3":dbl[](array[numeric])
  out "Transition weights 2":i32[](array[numeric])
  out "Position weights 2":i32[](array[numeric])
  out "averaged transition weights 2":dbl[](array[numeric])
  out "averaged position weights 2":dbl[](array[numeric])
  out "averaged position weights":dbl[](array[numeric])
  out "averaged transition weights":dbl[](array[numeric])
  out "Position weights":i32[](array[numeric])
  out "Transition weights":i32[](array[numeric])
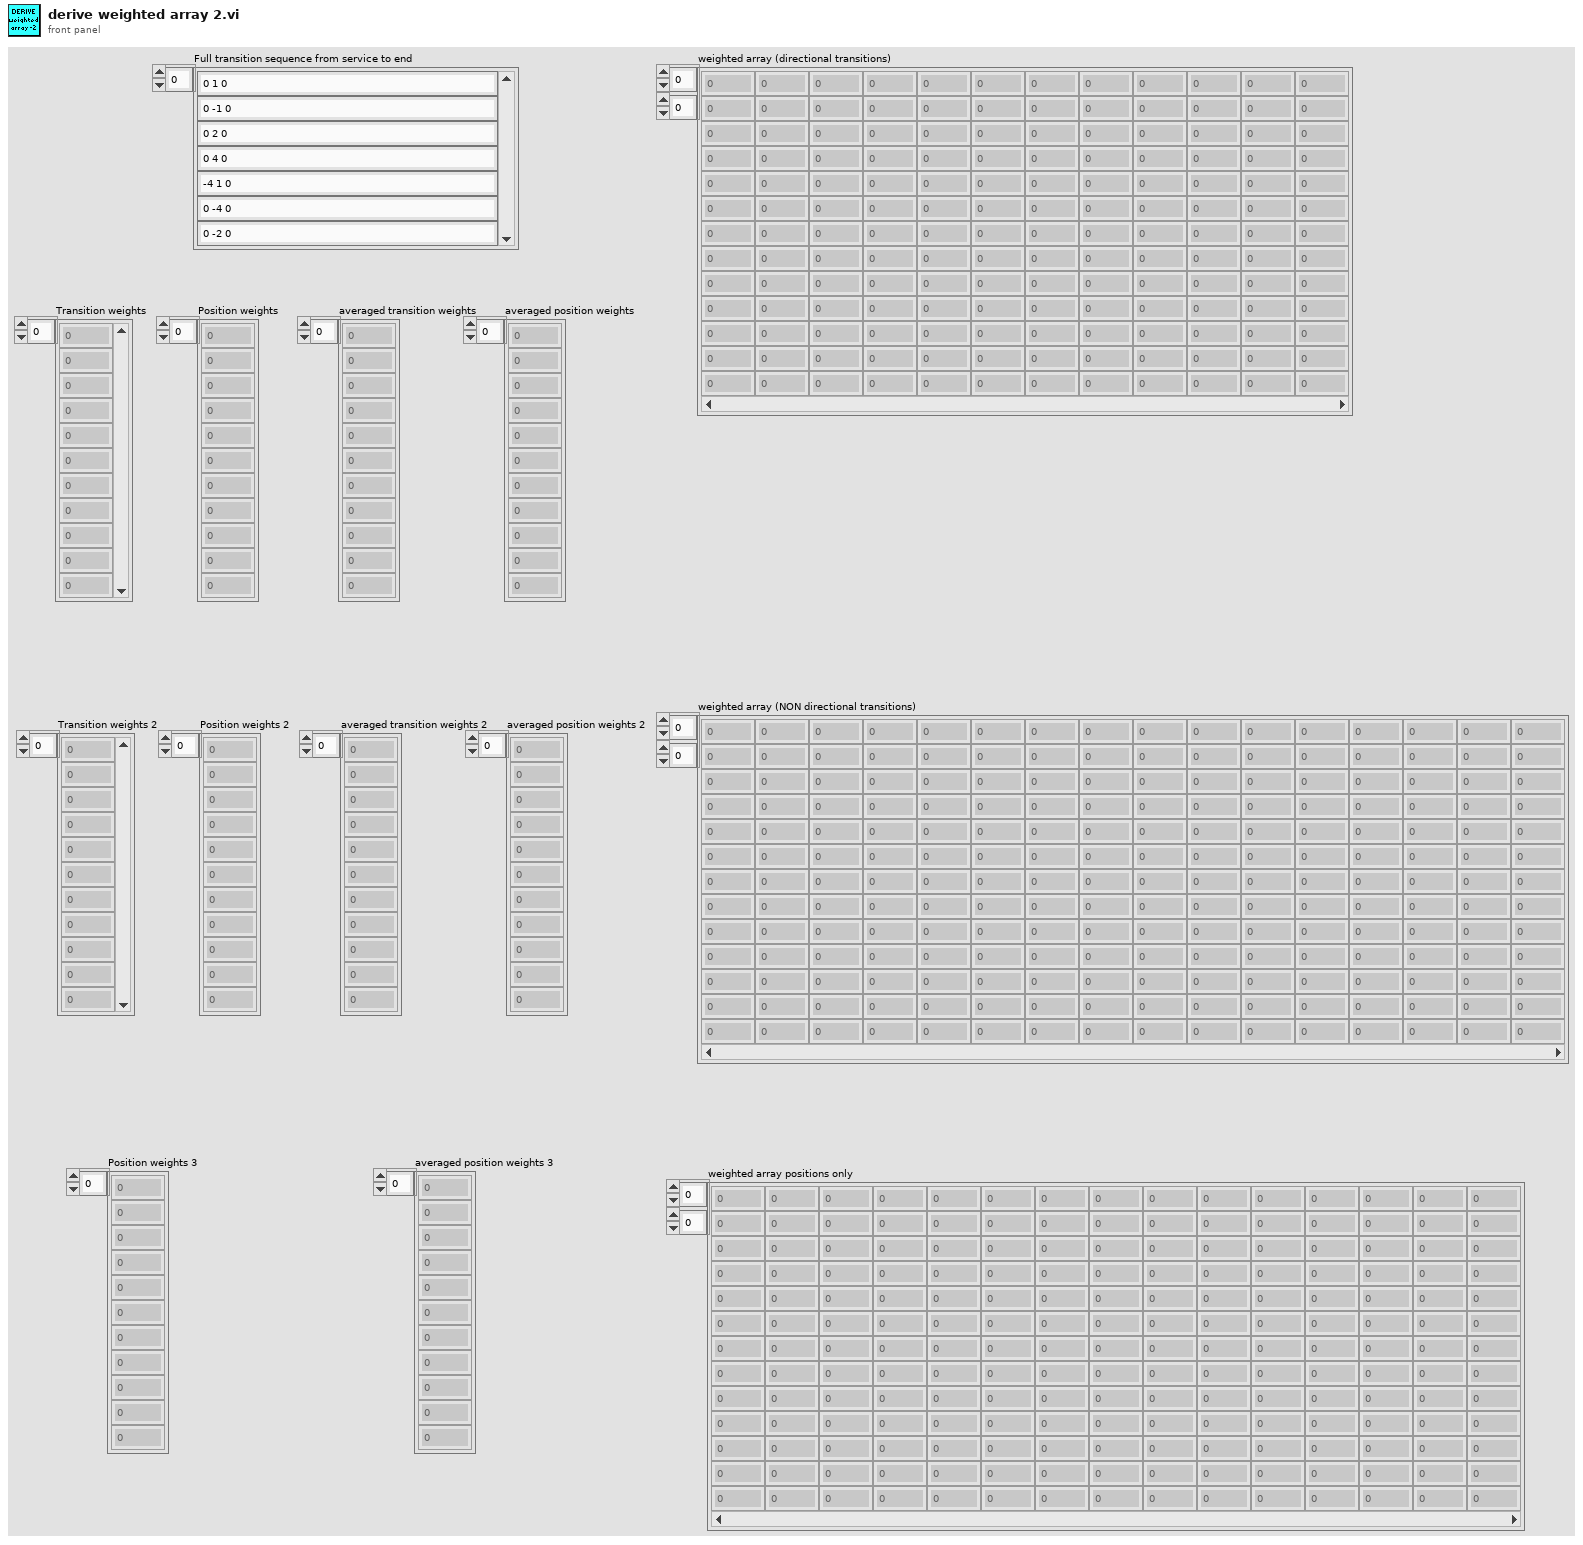
[diagram p1: front panel]
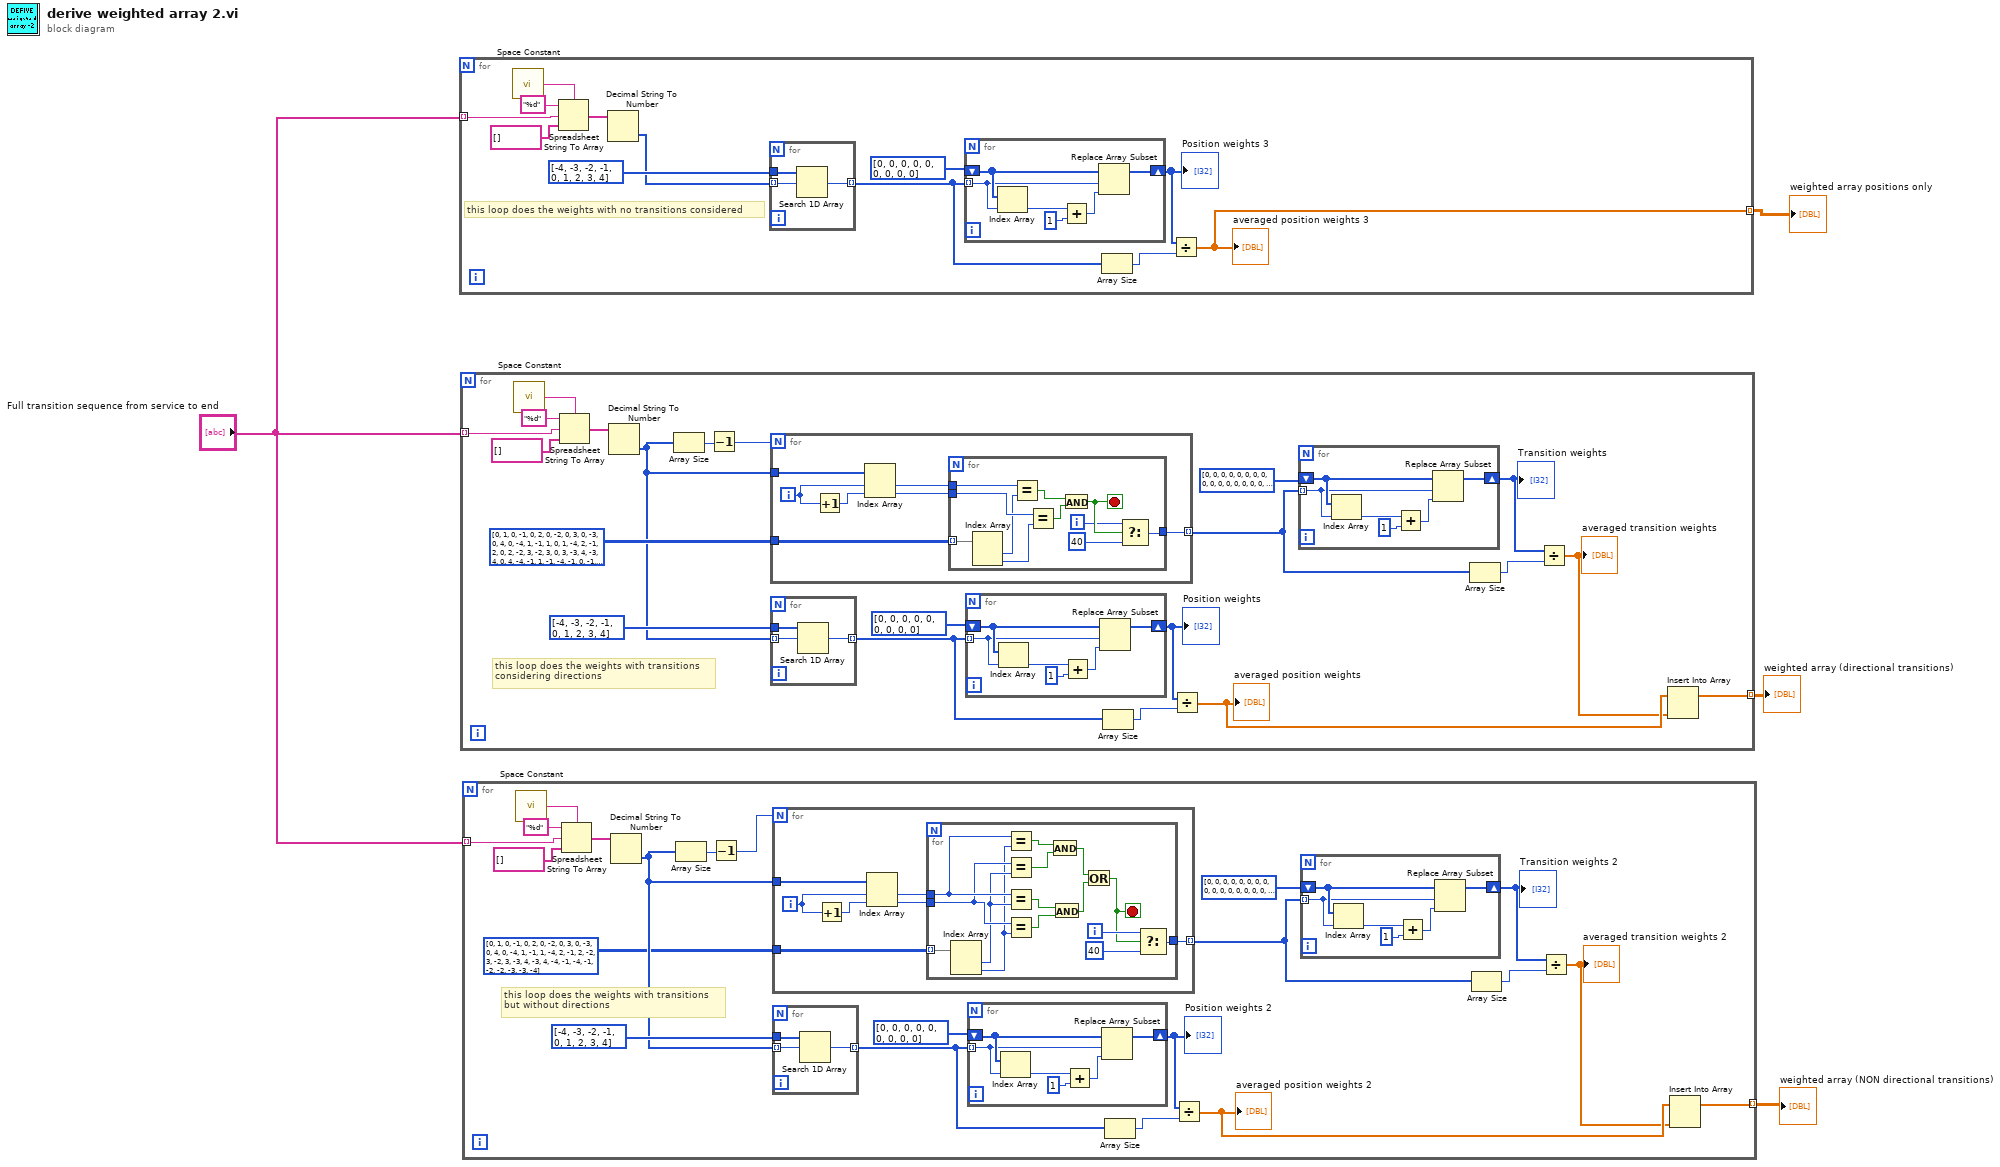
[diagram p0: block diagram]
diagram:
  n1 = for {
    tunnel: "Full transition sequence from service to end" -> [w12] mode=indexing
    tunnel: [w5] -> w1 mode=indexing
    # "this loop does the weights with no transitions considered"
    n2 = call <vilib>:"Space Constant.vi"() -> ("String"=w16:string)
    n3 = Spreadsheet String To Array(delimiter (Tab)=w16, format string="%d", spreadsheet string=w12, array type (2D Dbl)=string[] []) -> (array=w13:string[])
    n4 = Decimal String To Number(string=w13) -> (number=w10:i32[])  [unwired: 2 in, 1 out]
    n5 = for {
      tunnel: i32[] [-4, -3, -2, -1, 0, 1, 2, 3, 4] ("deleted portion") -> [w25]
      tunnel: w10 -> [w24] mode=indexing
      tunnel: [w23] -> w6 mode=indexing
      n6 = Search 1D Array(1D array=w25, element=w24) -> (index of element=w23:i32)  [unwired: 1 in]
    }
    n7 = for {
      tunnel: w6 -> [w19] mode=indexing
      shift-right: [w17] -> w7
      shift-left: i32[] [0, 0, 0, 0, 0, 0, 0, 0, 0] ("deleted portion") -> [w20]
      n8 = Index Array(array=w20, index=w19) -> (element=w22:i32)
      n9 = Add(x=w22, y=1) -> (x+y=w18:i32)
      n10 = Replace Array Subset(array=w20, new element=w18, index=w19) -> (w17:i32[])
    }
    "Position weights 3" <- w7
    n11 = Array Size(array=w6) -> (size(s)=w8:i32)
    n12 = Divide(x=w7, y=w8) -> (x/y=w5:dbl[])
    "averaged position weights 3" <- w5
  }
  "weighted array positions only" <- w1
  n13 = for {
    tunnel: "Full transition sequence from service to end" -> [w40] mode=indexing
    tunnel: [w26] -> w4 mode=indexing
    # "this loop does the weights with transitions\nconsidering directions"
    n14 = call <vilib>:"Space Constant.vi"() -> ("String"=w46:string)
    n15 = Spreadsheet String To Array(delimiter (Tab)=w46, format string="%d", spreadsheet string=w40, array type (2D Dbl)=string[] []) -> (array=w43:string[])
    n16 = Decimal String To Number(string=w43) -> (number=w36:i32[])  [unwired: 2 in, 1 out]
    n17 = Array Size(array=w36) -> (size(s)=w42:i32)
    n18 = Decrement(x=w42) -> (x-1=w41:i32)
    n19 = for {
      N: w41 -> [_]
      tunnel: w36 -> [w67]
      tunnel: i32[][] [[0, 1], [0, -1], [0, 2], [0, -2], [0, 3], [0, -3], [0, 4], [0, -4], [1, -1], [1, 0], [1, -4], [2, -1], [2, 0], [2, -2], [3, -2], [3, 0], [3, -3], [4, -3], [4, 0], [4, -4], [-1, 1], [-1, -4], [-1, 0], [-1, -2], [-1, 2], [-2, 2], [-2, -1], [-2, 0], [-2, -3], [-2, 3], [-3, 3], [-3, -2], [-3, 0], [-3, -4], [-3, 4], [-4, 4], [-4, -3], [-4, 0], [-4, -1], [-4, 1]] -> [w68]
      tunnel: [w62] -> w34 mode=indexing
      i -> [w66]
      n20 = Increment(x=w66) -> (x+1=w65:i32)
      n21 = Index Array(array=w67, index #1=w66, index #2=w65) -> (element #1=w64:i32, element #2=w63:i32)
      n22 = for {
        tunnel: w68 -> [w79] mode=indexing
        tunnel: w64 -> [w78]
        tunnel: w63 -> [w77]
        tunnel: [w69] -> w62
        i -> [w70]
        stop <- w72 stop-if-true
        n23 = Index Array(array=w79) -> (element #1=w76:i32, element #2=w75:i32)  [unwired: 2 in]
        n24 = Equal?(x=w78, y=w76) -> (x = y?=w74:bool)
        n25 = Equal?(x=w77, y=w75) -> (x = y?=w73:bool)
        n26 = And(x=w74, y=w73) -> (x .and. y?=w72:bool)
        n27 = Select(t=w70, s=w72, f=40) -> (s? t:f=w69:i32)
      }
    }
    n28 = for {
      tunnel: i32[] [-4, -3, -2, -1, 0, 1, 2, 3, 4] ("deleted portion") -> [w55]
      tunnel: w36 -> [w54] mode=indexing
      tunnel: [w53] -> w29 mode=indexing
      n29 = Search 1D Array(1D array=w55, element=w54) -> (index of element=w53:i32)  [unwired: 1 in]
    }
    n30 = for {
      tunnel: w29 -> [w49] mode=indexing
      shift-right: [w47] -> w30
      shift-left: i32[] [0, 0, 0, 0, 0, 0, 0, 0, 0] ("deleted portion") -> [w50]
      n31 = Index Array(array=w50, index=w49) -> (element=w52:i32)
      n32 = Add(x=w52, y=1) -> (x+y=w48:i32)
      n33 = Replace Array Subset(array=w50, new element=w48, index=w49) -> (w47:i32[])
    }
    "Position weights" <- w30
    n34 = Array Size(array=w29) -> (size(s)=w31:i32)
    n35 = Divide(x=w30, y=w31) -> (x/y=w28:dbl[])
    "averaged position weights" <- w28
    n36 = for {
      tunnel: w34 -> [w58] mode=indexing
      shift-right: [w56] -> w33
      shift-left: i32[] [0, 0, 0, 0, 0, 0, 0, 0, 0, 0, 0, 0, 0, 0, 0, 0, 0, 0, 0, 0, 0, 0, 0, 0, 0, 0, 0, 0, 0, 0, 0, 0, 0, 0, 0, 0, 0, 0, 0, 0] ("deleted portion") -> [w59]
      n37 = Index Array(array=w59, index=w58) -> (element=w61:i32)
      n38 = Add(x=w61, y=1) -> (x+y=w57:i32)
      n39 = Replace Array Subset(array=w59, new element=w57, index=w58) -> (w56:i32[])
    }
    "Transition weights" <- w33
    n40 = Array Size(array=w34) -> (size(s)=w32:i32)
    n41 = Divide(x=w33, y=w32) -> (x/y=w27:dbl[])
    "averaged transition weights" <- w27
    n42 = Insert Into Array(array=w28, new element=w27) -> (w26:dbl[])  [unwired: 1 in]
  }
  "weighted array (directional transitions)" <- w4
  n43 = for {
    tunnel: "Full transition sequence from service to end" -> [w94] mode=indexing
    tunnel: [w82] -> w3 mode=indexing
    # "this loop does the weights with transitions\nbut without directions"
    n44 = call <vilib>:"Space Constant.vi"() -> ("String"=w100:string)
    n45 = Spreadsheet String To Array(delimiter (Tab)=w100, format string="%d", spreadsheet string=w94, array type (2D Dbl)=string[] []) -> (array=w97:string[])
    n46 = Decimal String To Number(string=w97) -> (number=w92:i32[])  [unwired: 2 in, 1 out]
    n47 = Array Size(array=w92) -> (size(s)=w96:i32)
    n48 = Decrement(x=w96) -> (x-1=w95:i32)
    n49 = for {
      N: w95 -> [_]
      tunnel: w92 -> [w121]
      tunnel: i32[][] [[0, 1], [0, -1], [0, 2], [0, -2], [0, 3], [0, -3], [0, 4], [0, -4], [1, -1], [1, -4], [2, -1], [2, -2], [3, -2], [3, -3], [4, -3], [4, -4], [-1, -4], [-1, -2], [-2, -3], [-3, -4]] -> [w122]
      tunnel: [w116] -> w90 mode=indexing
      i -> [w120]
      n50 = Increment(x=w120) -> (x+1=w119:i32)
      n51 = Index Array(array=w121, index #1=w120, index #2=w119) -> (element #1=w118:i32, element #2=w117:i32)
      n52 = for {
        tunnel: w122 -> [w137] mode=indexing
        tunnel: w118 -> [w131]
        tunnel: w117 -> [w130]
        tunnel: [w132] -> w116
        i -> [w133]
        stop <- w123 stop-if-true
        n53 = Index Array(array=w137) -> (element #1=w129:i32, element #2=w128:i32)  [unwired: 2 in]
        n54 = Equal?(x=w131, y=w128) -> (x = y?=w127:bool)
        n55 = Equal?(x=w130, y=w129) -> (x = y?=w126:bool)
        n56 = Equal?(x=w131, y=w129) -> (x = y?=w136:bool)
        n57 = Equal?(x=w130, y=w128) -> (x = y?=w135:bool)
        n58 = And(x=w127, y=w126) -> (x .and. y?=w125:bool)
        n59 = And(x=w136, y=w135) -> (x .and. y?=w124:bool)
        n60 = Or(x=w125, y=w124) -> (x .or. y?=w123:bool)
        n61 = Select(t=w133, s=w123, f=40) -> (s? t:f=w132:i32)
      }
    }
    n62 = for {
      tunnel: i32[] [-4, -3, -2, -1, 0, 1, 2, 3, 4] ("deleted portion") -> [w109]
      tunnel: w92 -> [w108] mode=indexing
      tunnel: [w107] -> w85 mode=indexing
      n63 = Search 1D Array(1D array=w109, element=w108) -> (index of element=w107:i32)  [unwired: 1 in]
    }
    n64 = for {
      tunnel: w85 -> [w103] mode=indexing
      shift-right: [w101] -> w86
      shift-left: i32[] [0, 0, 0, 0, 0, 0, 0, 0, 0] ("deleted portion") -> [w104]
      n65 = Index Array(array=w104, index=w103) -> (element=w106:i32)
      n66 = Add(x=w106, y=1) -> (x+y=w102:i32)
      n67 = Replace Array Subset(array=w104, new element=w102, index=w103) -> (w101:i32[])
    }
    "Position weights 2" <- w86
    n68 = Array Size(array=w85) -> (size(s)=w87:i32)
    n69 = Divide(x=w86, y=w87) -> (x/y=w84:dbl[])
    "averaged position weights 2" <- w84
    n70 = for {
      tunnel: w90 -> [w112] mode=indexing
      shift-right: [w110] -> w89
      shift-left: i32[] [0, 0, 0, 0, 0, 0, 0, 0, 0, 0, 0, 0, 0, 0, 0, 0, 0, 0, 0, 0] ("deleted portion") -> [w113]
      n71 = Index Array(array=w113, index=w112) -> (element=w115:i32)
      n72 = Add(x=w115, y=1) -> (x+y=w111:i32)
      n73 = Replace Array Subset(array=w113, new element=w111, index=w112) -> (w110:i32[])
    }
    "Transition weights 2" <- w89
    n74 = Array Size(array=w90) -> (size(s)=w88:i32)
    n75 = Divide(x=w89, y=w88) -> (x/y=w83:dbl[])
    "averaged transition weights 2" <- w83
    n76 = Insert Into Array(array=w84, new element=w83) -> (w82:dbl[])  [unwired: 1 in]
  }
  "weighted array (NON directional transitions)" <- w3
